vi "Image Clustering.vi"(6 "Color Array":T1[](array[typedef]), 8 "Reflect":dbl[](array[numeric]), 9 "Z":dbl[](array[numeric]), 10 "Y":dbl[](array[numeric]), 11 "X":dbl[](array[numeric])) -> (0 "Indicies":u32[](array[numeric]), 1 "Colour Coords":T1[](array[typedef]), 2 "XYZ Coords":cluster{"X":dbl, "Y":dbl, "Z":dbl}[](array[cluster]))   [LabVIEW 2017]
uses:
  <vilib>/Utility/miscctls.llb/LVRGBAColorTypeDef.ctl
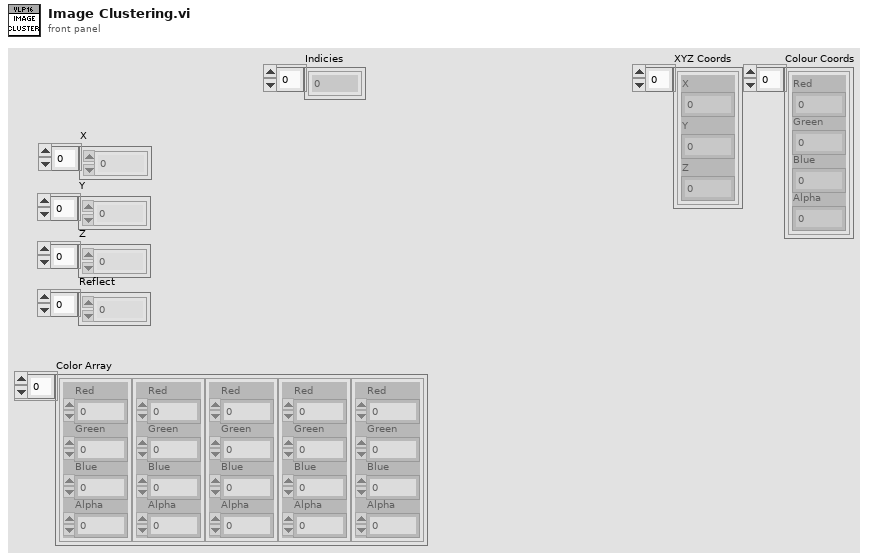
[diagram p1: front panel]
types:
  T1 = typedef "LVRGBAColorTypeDef.ctl" = cluster{"Red":sgl, "Green":sgl, "Blue":sgl, "Alpha":sgl}
  T2 = cluster{"Numeric":dbl, "Numeric":dbl, "Numeric":dbl}
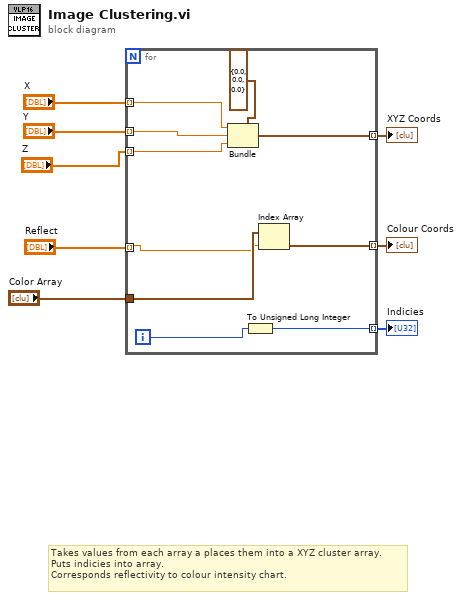
[diagram p0: block diagram]
diagram:
  # "Takes values from each array a places them into a XYZ cluster array.\nPuts indicies into array.\nCorresponds reflectivity to colour intensity chart."
  n1 = for {
    tunnel: "X" -> [w18] mode=indexing
    tunnel: "Y" -> [w17] mode=indexing
    tunnel: "Z" -> [w10] mode=indexing
    tunnel: [w15] -> w5 mode=indexing
    tunnel: "Color Array" -> [w14]
    tunnel: "Reflect" -> [w9] mode=indexing
    tunnel: [w13] -> w2 mode=indexing
    tunnel: [w11] -> w1 mode=indexing
    i -> [w12]
    n2 = Bundle(cluster=T2 {"Numeric"=0.0, "Numeric"=0.0, "Numeric"=0.0}, "Numeric"=w18, "Numeric"=w17, "Numeric"=w10) -> (w15:T2)
    n3 = To Unsigned Long Integer(number=w12) -> (unsigned 32bit integer=w11:u32)
    n4 = Index Array(array=w14, index=w9) -> (element=w13:T1)
  }
  "XYZ Coords" <- w5
  "Colour Coords" <- w2
  "Indicies" <- w1
